vi "GET NPSV URLs.vi"(8 "error in (no error)":errorcluster, 10 "Page":string, 11 "Device Reference in":T1 format="%.0x") -> (0 "error out":errorcluster, 1 "SV":T2, 2 "Channel Refs":T1[](array[typedef]) format="%.0x", 3 "Device Reference out":T1=18446744073709551615 format="%.0x")   [LabVIEW 2020, in "Shared Variables CD 2.0 Engine.lvlib"]
uses:
  Shared Variables CD 2.0 Engine.lvlib
  <vilib>/NI VeriStand/Custom Device API/Custom Device Item Ref.ctl
  Shared DataTypes/URLs.ctl
  <vilib>/Utility/error.llb/Error Cluster From Error Code.vi
  Shared/SV Global.vi
  <vilib>/ErrorRing/Error Ring.xnode
  <vilib>/NI VeriStand/Custom Device API/Custom Device API.lvlib
  <vilib>/NI VeriStand/Custom Device Tools/Custom Device Utility Library/Custom Device Utility Library.lvlib
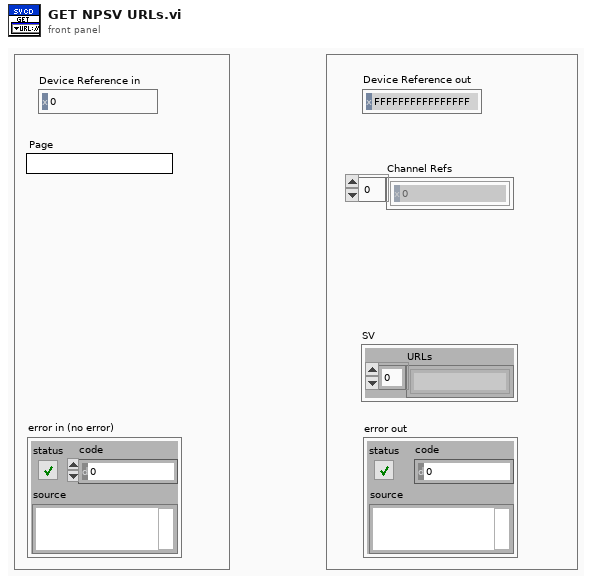
[diagram p1: front panel]
types:
  T1 = typedef "Custom Device API.lvlib/Custom Device Item Ref.ctl" = u64
  T2 = typedef "URLs.ctl" = cluster{"URLs":string[]}
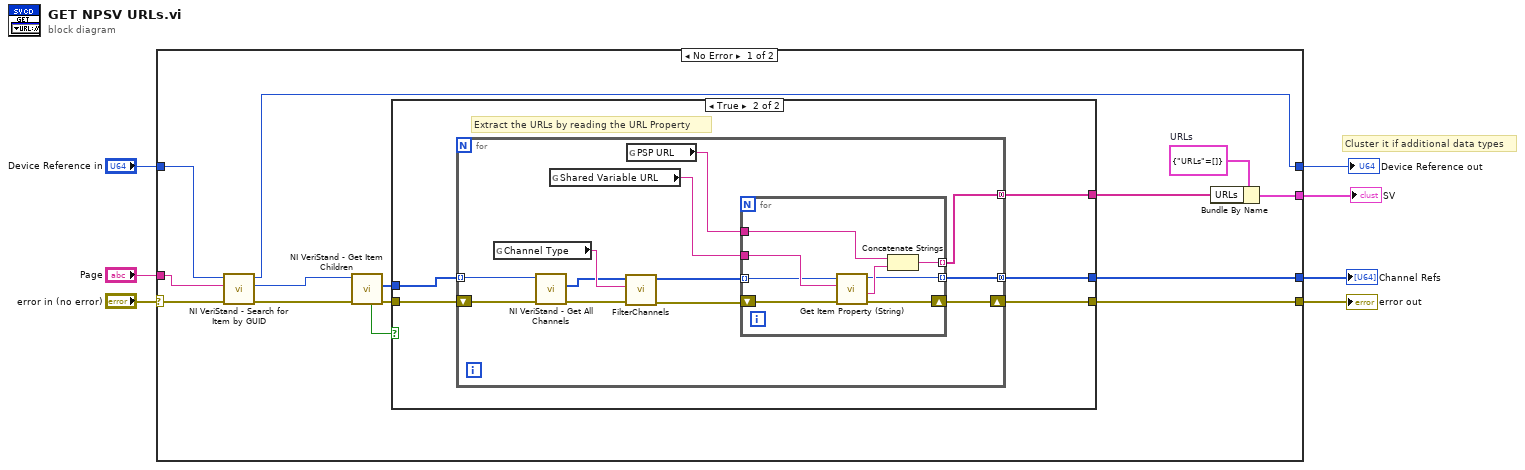
[diagram p0: block diagram]
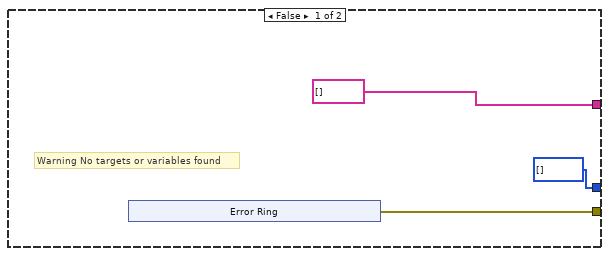
[diagram p2: hidden frame]
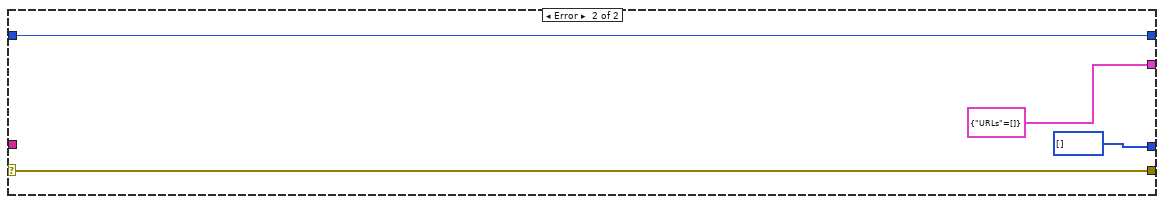
[diagram p3: hidden frame]
diagram:
  # "Cluster it if additional data types"
  n1 = case shown="No Error" "error in (no error)" {
    selector: "error in (no error)" -> [w12 w57]
    tunnel: [w21 w57] -> w7
    tunnel: "Device Reference in" -> [w20 w58]
    tunnel: "Page" -> [w14 _]
    tunnel: [w13 w58] -> w4
    tunnel: [w9 T2 {"URLs"=[]} ("URLs")] -> w2
    tunnel: [w8 T1[] [] ("Channel Refs")] -> w1
    frame No Error {
      w11 = T2 {"URLs"=[]}  # URLs
      n2 = call <vilib>:"NI VeriStand - Search for Item by GUID.vi"("error in"=w12, "Item GUID"=w14, "Section Ref in"=w20) -> ("error out"=w19:errorcluster, "Item Ref"=w15:T1, "Section Ref out"=w13:T1)  [unwired: 5 in, 1 out]
      n3 = call <vilib>:"NI VeriStand - Get Item Children.vi"("error in (no error)"=w19, "Item Ref in"=w15) -> ("error out"=w18:errorcluster, "Child Refs"=w16:T1[], "Found"=w17:bool)  [unwired: 6 in, 1 out]
      n4 = case shown="True" w17 {
        tunnel: w16 -> [_ w34]
        tunnel: w18 -> [_ w33]
        tunnel: [w24 w32] -> w21
        tunnel: [string[] [] w31] -> w10
        tunnel: [T1[] [] ("Channel Refs") w30] -> w8
        frame False {
          # "Warning No targets or variables found"
          n5 = xnode "Error Ring"() -> ("error out"=w24:errorcluster)
        }
        frame True {
          # "Extract the URLs by reading the URL Property"
          n6 = for {
            tunnel: w34 -> [w46] mode=indexing
            shift-right: [w38] -> w32
            shift-left: w33 -> [w45]
            tunnel: [w39] -> w31 mode=concatenating
            tunnel: [w35] -> w30 mode=concatenating
            n7 = global read "SV Global.vi" "Channel Type"() -> (w44:string)
            n8 = call <vilib>:"NI VeriStand - Get All Channels.vi"("error in"=w45, "Section Ref in"=w46) -> ("error out"=w43:errorcluster, "Channel Refs"=w37:T1[])  [unwired: 6 in, 2 out]
            n9 = global read "SV Global.vi" "Shared Variable URL"() -> (w40:string)
            n10 = call "FilterChannels.vi"("error in (no error)"=w43, "Property"=w44, "Specified Channel Ref List"=w37) -> ("error out"=w42:errorcluster, "Filtered Channel list"=w36:T1[])  [unwired: 7 in]
            n11 = global read "SV Global.vi" "PSP URL"() -> (w41:string)
            n12 = for {
              tunnel: w41 -> [w51]
              shift-right: [w53] -> w38
              shift-left: w42 -> [w54]
              tunnel: w40 -> [w52]
              tunnel: [w50] -> w39 mode=indexing
              tunnel: w36 -> [w48] mode=indexing
              tunnel: [w47] -> w35 mode=indexing
              n13 = call <vilib>:"Get Item Property (String).vi"("error in (no error)"=w54, "Property Name"=w52, "Item Ref in"=w48) -> ("error out"=w53:errorcluster, "Value"=w49:string, "Item Ref out"=w47:T1)  [unwired: 5 in, 1 out]
              n14 = Concatenate Strings(w51, w49) -> (w50:string)
            }
          }
        }
      }
      n15 = Bundle By Name(cluster=w11, "URLs"=w10) -> (w9:T2)
    }
    frame Error {
    }
  }
  "error out" <- w7
  "Device Reference out" <- w4
  "SV" <- w2
  "Channel Refs" <- w1
